vi "PID control fhd.vi"() -> ()   [LabVIEW 2017]
uses:
  <vilib>/Simulation/Scripting/Companion Diagram/SimConfigNode/SimParams.ctl
  <vilib>/Simulation/Scripting/Companion Diagram/SimConfigNode/_simSolvers.ctl
  <vilib>/Simulation/Implementation/Shared/SIMSCR Execution Mode.ctl
  <vilib>/Simulation/Param Hierarchy/Typedefs/SIMPH Param Control Actions.ctl
  <vilib>/Simulation/Implementation/Shared/NILVSim_ParamChanged.vi
  <vilib>/Simulation/Implementation/Shared/NILVSIM_BeginStep.vi
  <vilib>/Simulation/Implementation/Shared/NILVSim_Manager.vi
  <vilib>/Utility/error.llb/Clear Errors.vi
  <vilib>/Simulation/Implementation/Shared/NILVSim_FinalizeModel.vi
  <vilib>/DAQmx/read.llb/DAQmx Read (Counter DBL 1Chan 1Samp).vi
  <vilib>/DAQmx/read.llb/DAQmx Read (Digital Bool 1Line 1Point).vi
  917b7e52-755f-4d44-bea8-9e7c9beac24e.vi
  a58f9967-76f1-4ebc-ad3d-26e75a3ca160.vi
  <vilib>/DAQmx/write.llb/DAQmx Write (Analog DBL 1Chan 1Samp).vi
  <vilib>/DAQmx/create/channels.llb/DAQmx Create Channel (AO-Voltage-Basic).vi
  <vilib>/DAQmx/create/channels.llb/DAQmx Create Channel (DI-Digital Input).vi
  <vilib>/DAQmx/create/channels.llb/DAQmx Create Channel (CI-Count Edges).vi
  <vilib>/Simulation/Implementation/Shared/SIM Unbundle Sim Info.vi
  <vilib>/Simulation/Implementation/Shared/NILVSim_Initialize.vi
  <vilib>/Simulation/Utility/Implementation/NILVSim Get Time and IsAcceptedStep.vi
  <vilib>/Simulation/Implementation/Shared/SIMSH Read Queue.vi
  <vilib>/Simulation/Implementation/Shared/NILVSim_GetModelError.vi
  <vilib>/Simulation/Implementation/Shared/SIM Bundle Sim Info.vi
  <vilib>/DAQmx/miscellaneous.llb/DAQmx Fill In Error Info.vi
  <vilib>/Simulation/Implementation/XNodeFramework/SimXNode/SimX.xnode
  <vilib>/Simulation/Model Libraries/PID/SIM PID (Parallel).vi
  <vilib>/Simulation/Model Libraries/PID/SIM PID.vi
  <vilib>/Simulation/Scripting/Companion Diagram/SimConfigNode/SimDog.xnode
  <vilib>/Simulation/Model Libraries/PID/SIM PID (Academic).vi
  <vilib>/Simulation/Implementation/Shared/NI_SIM_Implementation.lvlib
panel:
  out "Error in x direction":dbl
  out "Error in y direction":dbl
  out "Yerror":dbl
  out "Xerror":dbl
  out "Boolean":bool
  out "Numeric 3":dbl
  out "variable to stop":dbl
  out "index":dbl
  out "x check":dbl
  out "stop":bool
  out "y final check":dbl
  out "y check":dbl
  out "array x Length":dbl
  out "X array":dbl[](array[numeric])
  out "array Y length":dbl
  out "Y array":dbl[](array[numeric])
  out "Numeric y":dbl
  out "Numeric x":dbl
  out "Numeric 2":dbl
  in  "Radius":dbl
  out "led check":bool
  in  "check instruc":bool
  out "down 2":bool
  out "down":bool
  out "right":bool
  out "x entered":dbl
  out "y enetred":dbl
  out "greater -1 x":bool
  out "less 1 x":bool
  out "direction selected":dbl
  out "circle reset":bool
  in  "part circle":T1(ring)=enum."a"
  out "at 2f":bool
  out "Step 2J":bool
  out "Step 2H":bool
  out "Shape drawing steps":enum16{"corner", "1st switch", "reverse"}(ring)
  out "Step 2D":bool
  out "Step 2C":bool
  out "c":bool
  in  "height":dbl
  in  "length":dbl
  in  "part":T2(ring)=enum."a"
  out "Step 2A":bool
  out "Step 2B":bool
  in  "Has encoders been reset?":enum16{"don't reset", "reset"}(ring)
  out "x distance currently being travelled":dbl
  out "y distance currently being travelled":dbl
  out "error calced":dbl
  out "p1 dis 2":dbl
  out "p1 dis":dbl
  out "error y":dbl
  out "calc distance y":dbl
  out "calc distanc x":dbl
  out "error x":dbl
  out "reached y":bool
  out "reached x":bool
  out "Numeric":dbl
  in  "Draw rectangle":bool
  in  "Draw circle":bool
  out "In drawing mode":bool
  in  "Right-Down":bool
  in  "Left-Up":bool
  in  "Left-Down":bool
  in  "Right-Up":bool
  in  "right":bool
  in  "left":bool
  in  "motor 2":dbl(slide)=1.5 scale=-10.0..10.0
  in  "down":bool
  in  "up":bool
  in  "Y Length":dbl=30.0
  in  "X Length":dbl=30.0
  in  "Motor 2 encoder":tag="Dev1/ctr1"
  out "Pulses M2":dbl format="%.2f"
  in  "Motor 1 encoder":tag="Dev1/ctr0"
  out "Pulses M1":dbl format="%.2f"
  out "Right":bool
  out "Bottom":bool
  out "Left":bool
  out "Top":bool
  in  "Switch 4/Line 3":tag="Dev1/port0/line3"
  in  "Switch 3/Line 2":tag="Dev1/port0/line2"
  in  "Switch 2/Line 1":tag="Dev1/port0/line1"
  in  "Switch 1/Line 0":tag="Dev1/port0/line0"
  in  "Motor stop":bool
  in  "Motor 1":tag="Dev1/ao0"
  in  "max Voltage":dbl=10.0
  in  "Min Voltage":dbl=-10.0
  in  "Motor 2":tag="Dev1/ao1"
  in  "motor 1":dbl(slide)=1.5 scale=-10.0..10.0
  in  "stop":bool
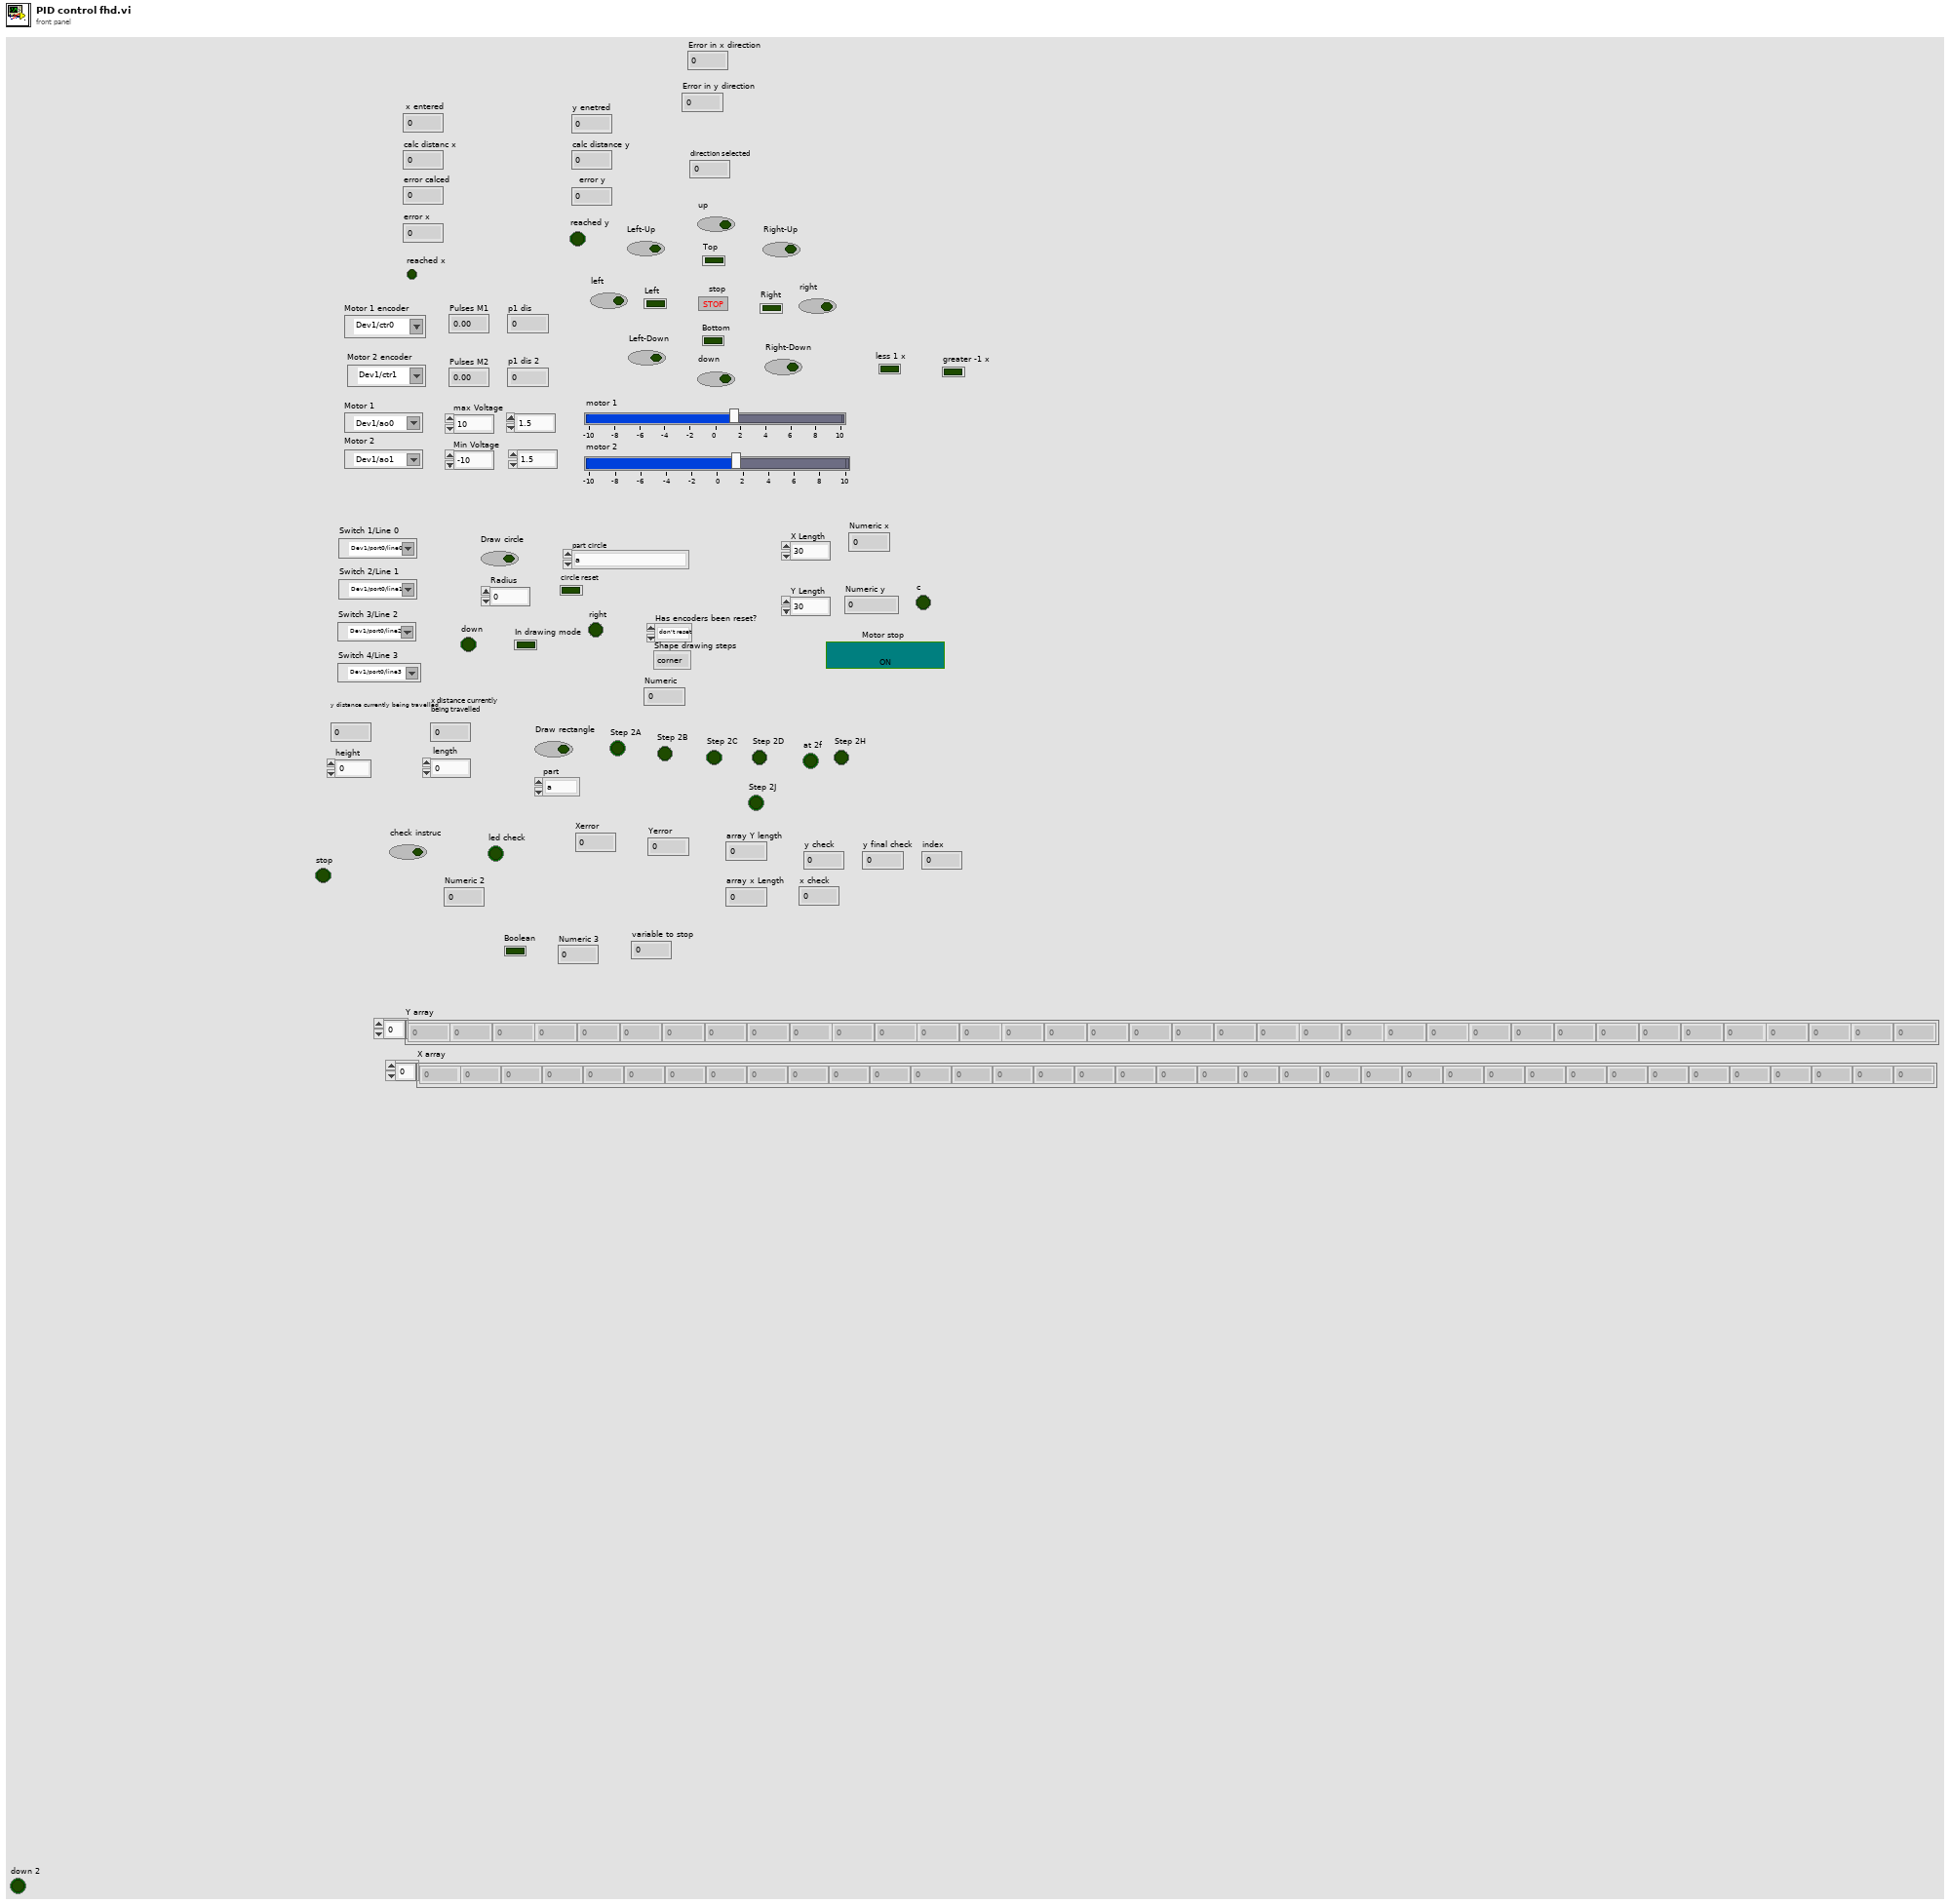
[diagram p1: front panel]
types:
  T1 = enum16{"nothing", "circle", "reset_before_circle", "radius_travel", "going right", "going down", "a"}
  T2 = enum16{"nothing", "j", "i", "h", "g", "f", "e", "d", "c", "b", "a"}
  T3 = enum16{"Simulate to Completion", "Single Time-Step Simulation (Fixed Step Only)"}
  T4 = typedef "SIMSCR Execution Mode.ctl" = enum16{"Simulate to Completion", "Single Time-Step Simulation (Fixed Step Only)"}
  T5 = typedef "SIMPH Param Control Actions.ctl" = enum16{"get params", "set params"}
  T6 = cluster{"SIMSH Sim Time":dbl, "SIM PID Derivative Gain.vi":cluster{"output":dbl}, "SIM PID Derivative Gain.vi - SIMSH":cluster{"SIMSH Sim Time":dbl, "t 3":dbl, "Select 2":cluster{"s? t:f":dbl}, "Equal?":cluster{"x = y?":bool}, "Or":cluster{"x .or. y?":bool}, "Equal To 0?":cluster{"x = 0?":bool}}, "High Frequency [s] (Tf)":dbl, "Gain":cluster{"output":dbl}, "Summation":cluster{"Result":dbl}, "Integral Gain - series.vi":cluster{"output":dbl}, "Integral Gain - series.vi - SIMSH":cluster{"SIMSH Sim Time":dbl, "Select 2":cluster{"s? t:f":dbl}, "integral in gain?":bool, "Integrator":cluster{"output y(t)":dbl}, "Gain 2":cluster{"output":dbl}, "Select":cluster{"s? t:f":dbl}, "Equal To 0?":cluster{"x = 0?":bool}, "Reciprocal":cluster{"1/x":dbl}}}
  T7 = typedef "SimParams.ctl" = cluster{"Initial Time (s)":dbl, "Final Time (s)":dbl, "Step Size (s)":dbl, "ODE Solver":T8, "Minimum Step Size (s)":dbl, "Maximum Step Size (s)":dbl, "Relative Tolerance":dbl, "Absolute Tolerance":dbl, "Software Timing":bool, "Initial Step Size (s)":dbl, "Automatic Fixed Step Size?":bool, "Automatic Discrete Step Size?":bool, "Discrete Step Size (s)":dbl, "Calculate using Time Step":bool, "Solver Wired?":bool, "Prev.Frm.Expected End":u64, "Prev.Frm.Actual End":u64, "Prev.Frm.Finished Late?":bool, "Prev.Iter.Expected End":u64, "Prev.Iter.Actual End":u64, "Prev.Iter.Finished Late?":bool, "Expected Iteration Start":u64, "Actual Iteration Start":u64, "Expected Frame Start":u64, "Actual Frame Start":u64, "Source Name":string, "Name":string, "Period":i64, "Deadline":i64, "Offset":i64, "Start":i64, "Priority":i32, "Timeout":i32, "Processor":i32, "Mode":enum32{"No Change", "Process missed periods, maintain original phase", "Discard missed periods, maintain original phase", "Process missed periods, ignore original phase", "Discard missed periods, ignore original phase"}, "Wakeup reason":enum32{"Normal", "Aborted", "Asynchronous wakeup", "Timing source error", "Timed loop error", "Timeout"}, "Error":errorcluster, "Source Type":string, "Secondary Source Type":string, "Global End Time":u64, "Global Start Time":u64, "Full Solver Reset":bool, "Execution Mode":T4, "Nan/Inf Check":bool, "Custom Solver Library":string, "Solver Is Variable":bool, "custom solver name":string, "Signal Collection Decimation":u32}
  T8 = typedef "_simSolvers.ctl" = enum16{"Runge-Kutta 1 (Euler)", "Runge-Kutta 2", "Runge-Kutta 3", "Runge-Kutta 4", "Runge-Kutta 23 (variable)", "Runge-Kutta 45 (variable)", "BDF (variable)", "Adams-Moulton (variable)", "Rosenbrock (variable)", "Discrete States Only", "SDIRK 4 (variable)", "Radau 5 (variable)", "Radau 9 (variable)", "Radau 13 (variable)", "Radau [Variable Order] (variable)", "Gear's Method (variable)", "Linearizer", "State Query", "Trim Eval", "Custom Solver"}
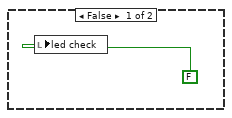
[diagram p2: hidden frame]
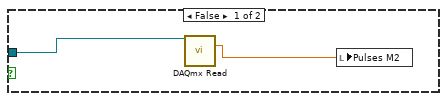
[diagram p3: hidden frame]
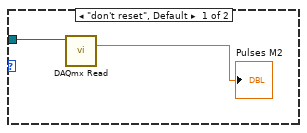
[diagram p4: hidden frame]
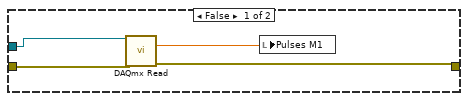
[diagram p5: hidden frame]
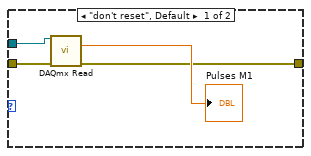
[diagram p6: hidden frame]
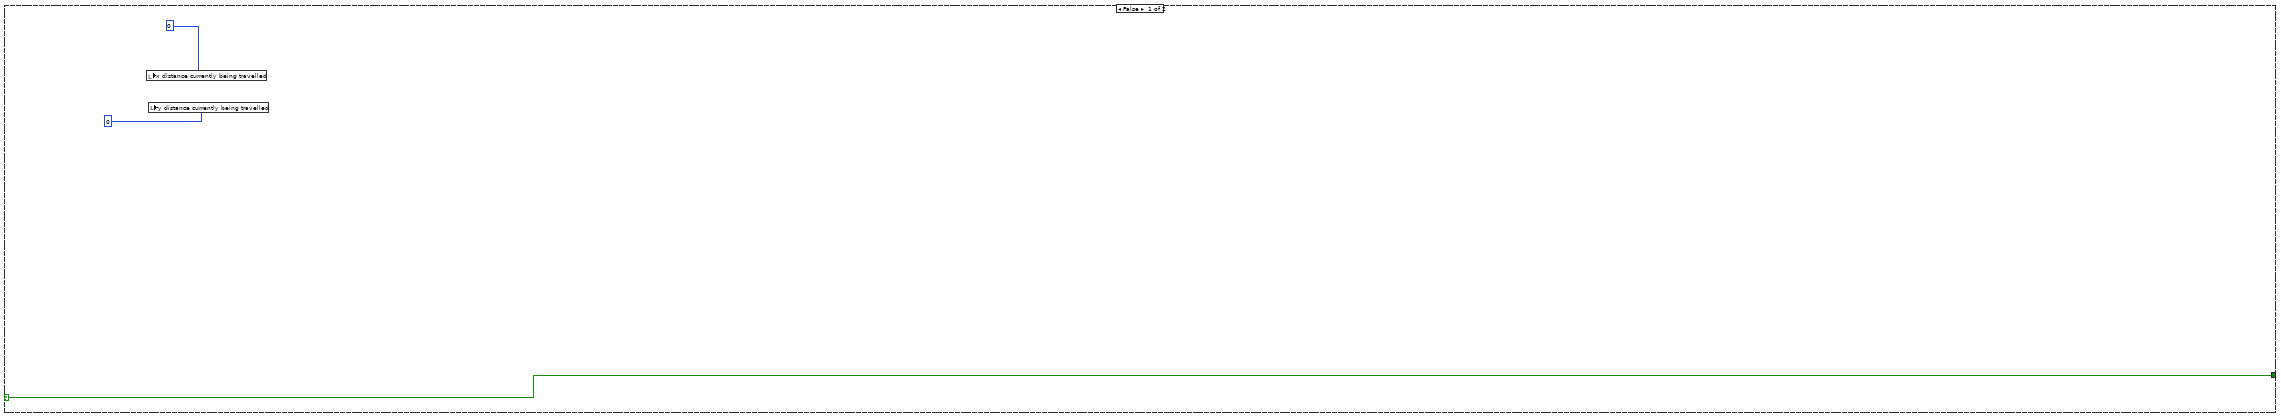
[diagram p7: hidden frame]
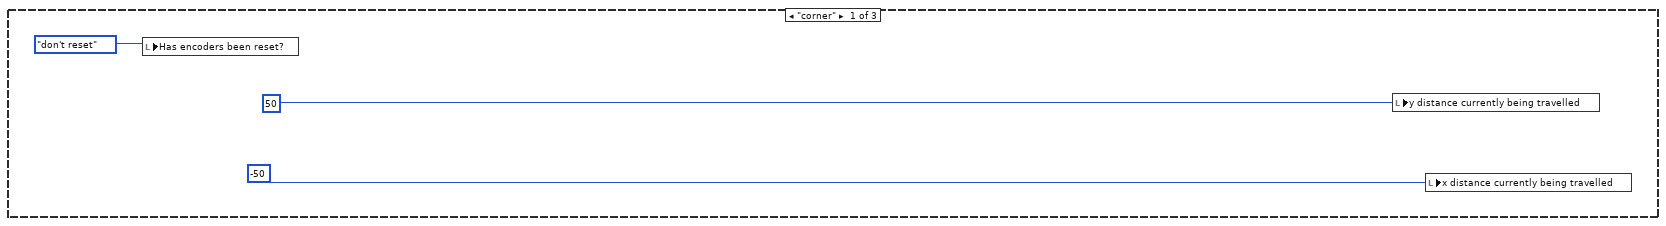
[diagram p8: hidden frame]
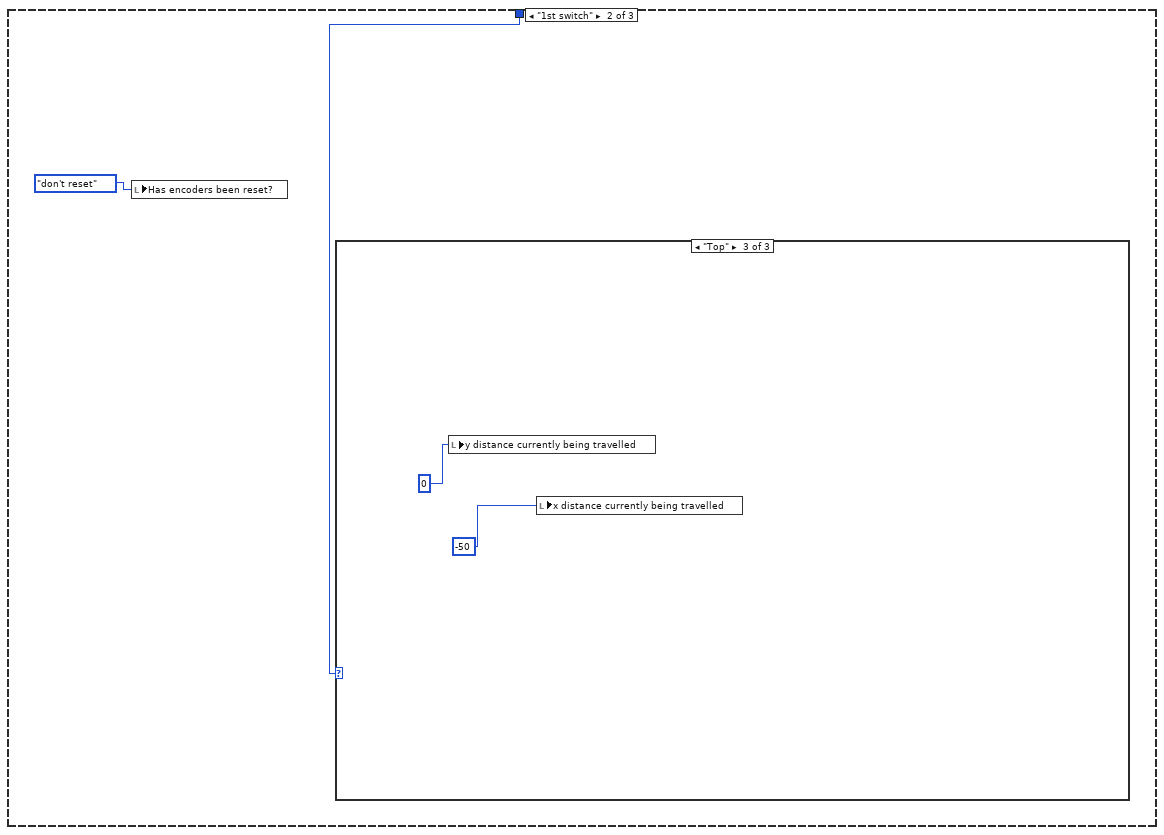
[diagram p9: hidden frame]
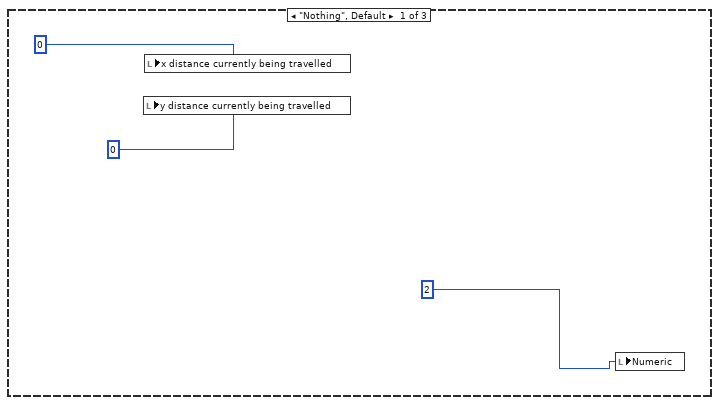
[diagram p10: hidden frame]
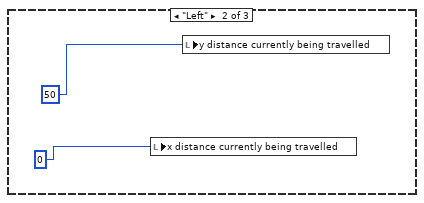
[diagram p11: hidden frame]
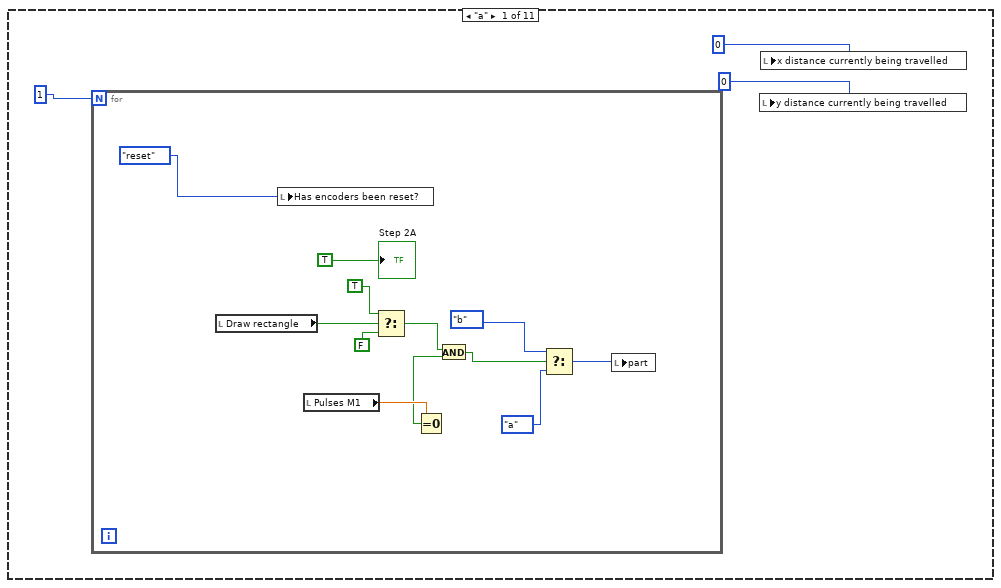
[diagram p12: hidden frame]
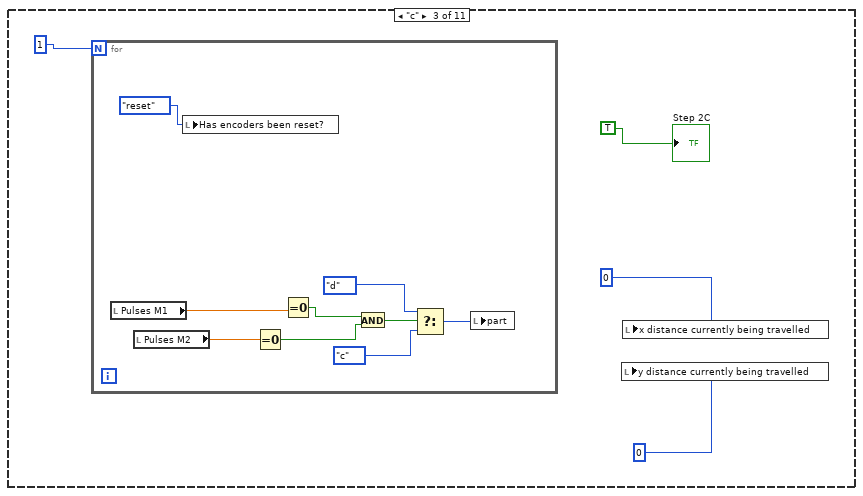
[diagram p13: hidden frame]
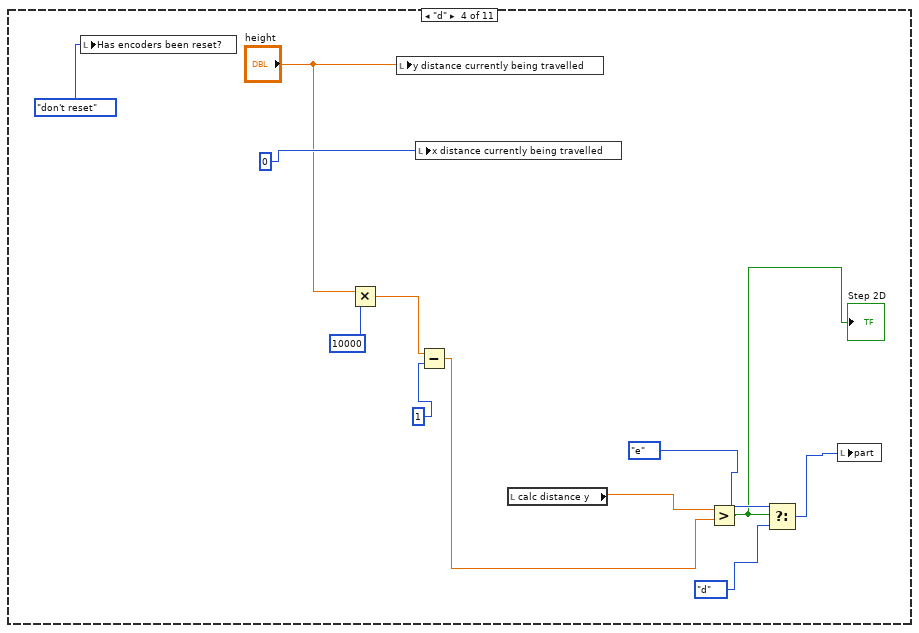
[diagram p14: hidden frame]
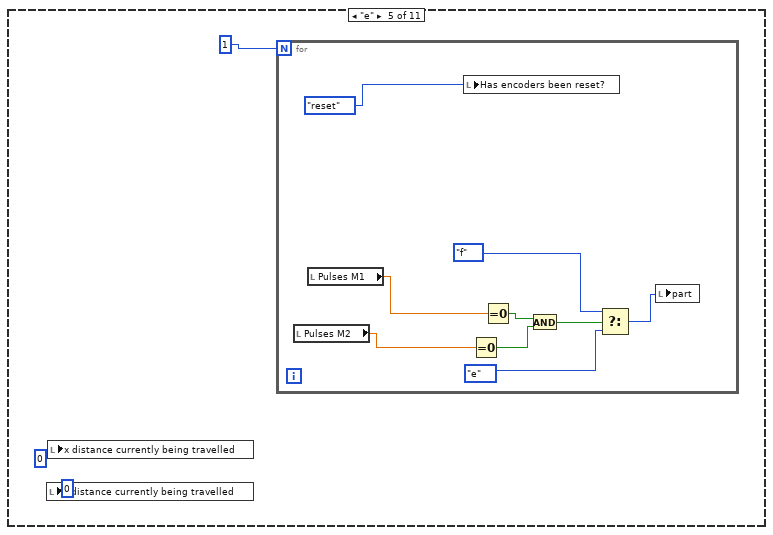
[diagram p15: hidden frame]
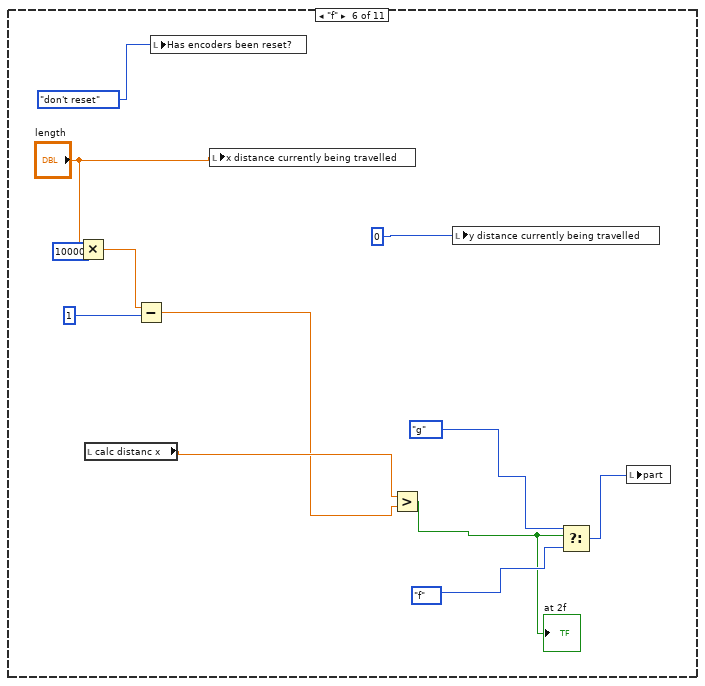
[diagram p16: hidden frame]
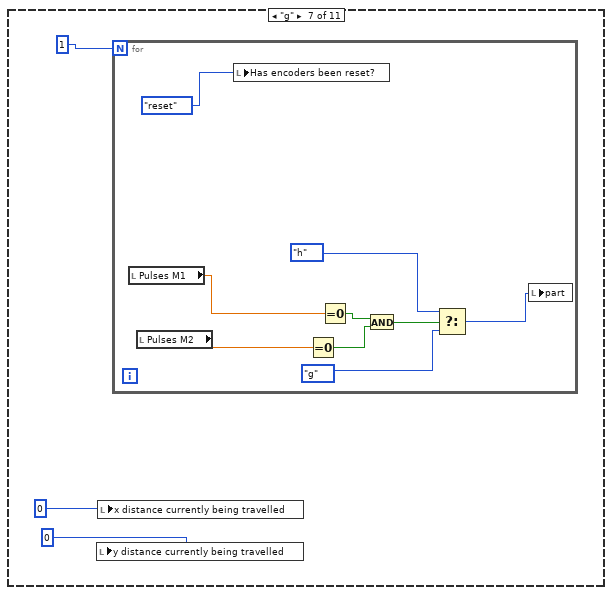
[diagram p17: hidden frame]
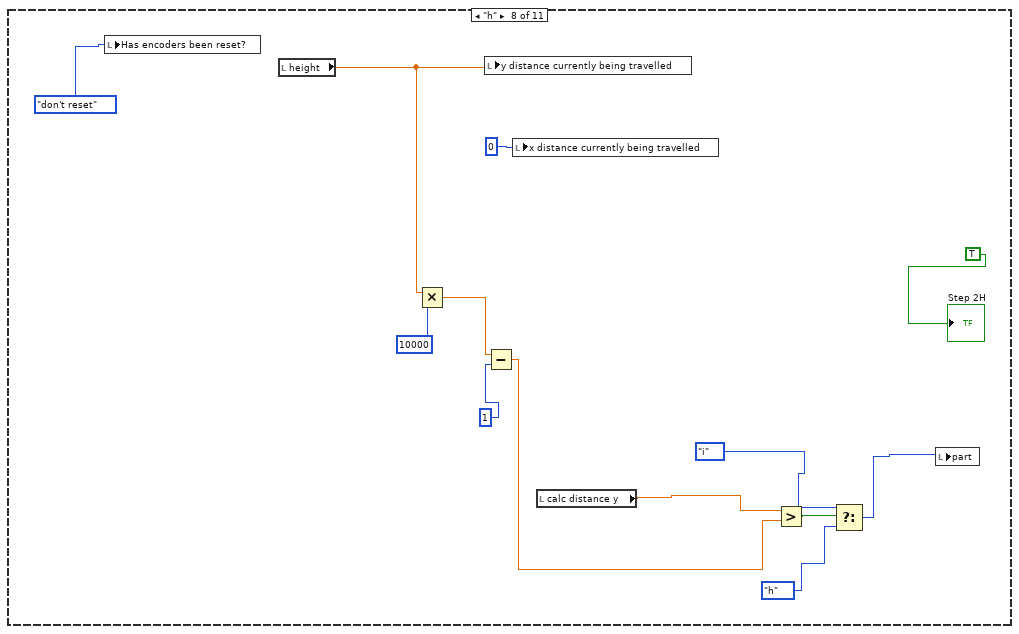
[diagram p18: hidden frame]
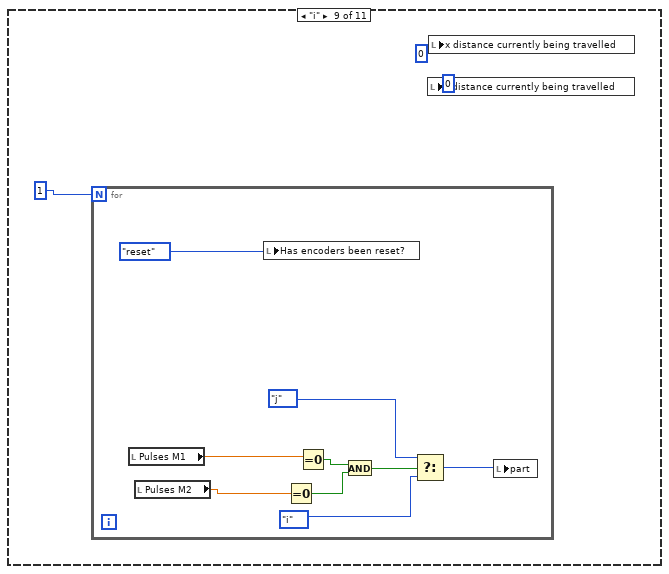
[diagram p19: hidden frame]
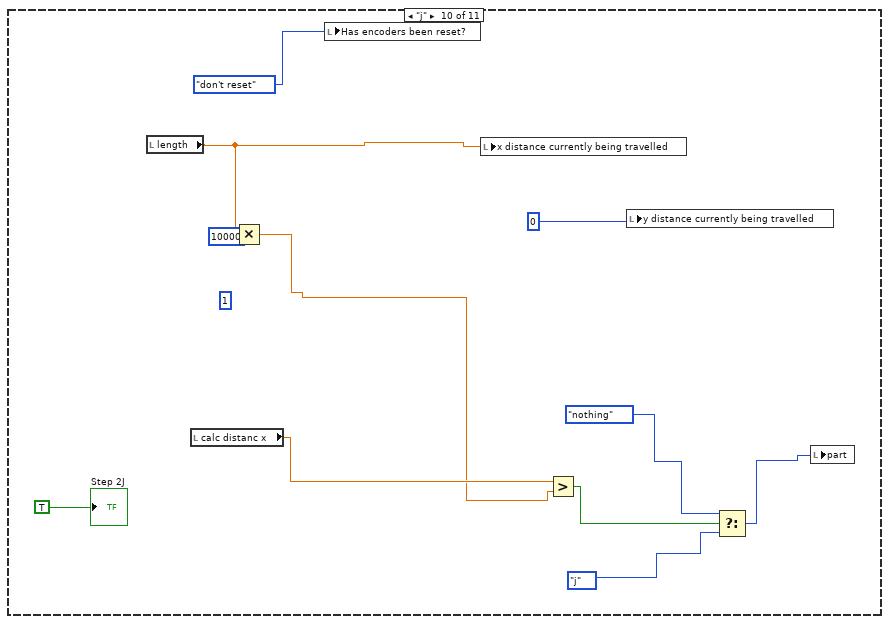
[diagram p20: hidden frame]
diagram:
  n1 = call-poly <vilib>:"DAQmx Create Virtual Channel.vi"("lines"="Switch 1/Line 0") -> ("task out"=w36:refnum<k21>, "error out"=w32:errorcluster)  [unwired: 13 in]
  n2 = call-poly <vilib>:"DAQmx Create Virtual Channel.vi"("lines"="Switch 2/Line 1") -> ("task out"=w35:refnum<k21>, "error out"=w31:errorcluster)  [unwired: 13 in]
  n3 = call-poly <vilib>:"DAQmx Create Virtual Channel.vi"("lines"="Switch 3/Line 2") -> ("task out"=w34:refnum<k21>, "error out"=w30:errorcluster)  [unwired: 13 in]
  n4 = call-poly <vilib>:"DAQmx Create Virtual Channel.vi"("lines"="Switch 4/Line 3") -> ("task out"=w33:refnum<k21>, "error out"=w29:errorcluster)  [unwired: 13 in]
  n5 = call <vilib>:"DAQmx Start Task.vi"("task/channels in"=w36, "error in"=w32) -> ("task out"=w28:refnum<k21>, "error out"=w26:errorcluster)  [unwired: 12 in]
  n6 = call <vilib>:"DAQmx Start Task.vi"("task/channels in"=w35, "error in"=w31) -> ("task out"=w24:refnum<k21>, "error out"=w21:errorcluster)  [unwired: 12 in]
  n7 = call <vilib>:"DAQmx Start Task.vi"("task/channels in"=w34, "error in"=w30) -> ("task out"=w23:refnum<k21>, "error out"=w20:errorcluster)  [unwired: 12 in]
  n8 = call <vilib>:"DAQmx Start Task.vi"("task/channels in"=w33, "error in"=w29) -> ("task out"=w22:refnum<k21>, "error out"=w19:errorcluster)  [unwired: 12 in]
  n9 = call-poly <vilib>:"DAQmx Create Virtual Channel.vi"("maximum value"="max Voltage", "minimum value"="Min Voltage", "physical channels"="Motor 1") -> ("task out"=w46:refnum<k21>, "error out"=w42:errorcluster)  [unwired: 11 in]
  n10 = call-poly <vilib>:"DAQmx Create Virtual Channel.vi"("counter"="Motor 2 encoder") -> ("task out"=w6:refnum<k21>)  [unwired: 13 in, 1 out]
  n11 = call-poly <vilib>:"DAQmx Create Virtual Channel.vi"("maximum value"="max Voltage", "minimum value"="Min Voltage", "physical channels"="Motor 2") -> ("task out"=w49:refnum<k21>, "error out"=w41:errorcluster)  [unwired: 11 in]
  n12 = call-poly <vilib>:"DAQmx Create Virtual Channel.vi"("counter"="Motor 1 encoder") -> ("task out"=w7:refnum<k21>, "error out"=w2:errorcluster)  [unwired: 13 in]
  n13 = call <vilib>:"DAQmx Start Task.vi"("task/channels in"=w6) -> ("task out"=w1:refnum<k21>)  [unwired: 13 in, 1 out]
  n14 = call <vilib>:"DAQmx Start Task.vi"("task/channels in"=w7) -> ("task out"=w3:refnum<k21>)  [unwired: 13 in, 1 out]
  n15 = while {
    tunnel: w49 -> [w228]
    tunnel: [w225] -> w48
    tunnel: w46 -> [w222]
    tunnel: [w221] -> w45
    tunnel: w42 -> [w219]
    tunnel: w41 -> [w218]
    tunnel: w28 -> [w212]
    tunnel: [w211] -> w27
    tunnel: w26 -> [w210]
    tunnel: [w209] -> w25
    tunnel: w24 -> [w208]
    tunnel: w23 -> [w207]
    tunnel: w22 -> [w206]
    tunnel: w21 -> [w205]
    tunnel: w20 -> [w204]
    tunnel: w19 -> [w203]
    tunnel: [w202] -> w18
    tunnel: [w201] -> w17
    tunnel: [w200] -> w16
    tunnel: [w199] -> w15
    tunnel: [w198] -> w14
    tunnel: [w197] -> w13
    tunnel: [w131] -> w10
    tunnel: w3 -> [w133]
    tunnel: w2 -> [w132]
    tunnel: w1 -> [w129]
    stop <- "stop" stop-if-true
    (unwired) TRUE
    n16 = Or(x="Draw circle", y="Draw rectangle") -> (x .or. y?=w141:bool)
    n17 = case shown="True" "check instruc" {
      frame False {
        n18 = local write "led check"(FALSE) -> ()
      }
      frame True {
        n19 = flat-sequence {
          frame #0 {
            n20 = while {
              stop <- w237 stop-if-true
              n21 = for {
                N: 50 -> [_]
                shift-right: [w243] -> w236
                shift-left: _ -> [_]
                tunnel: [w243] -> w231 mode=indexing
                shift-right: [w242] -> w234
                shift-left: _ -> [_]
                tunnel: [w242] -> w232 mode=indexing
                i -> [w245]
                n22 = Multiply(x=2, y=3.141592653589793) -> (x*y=w249:dbl)
                n23 = Increment(x=w245) -> (x+1=w247:i32)
                n24 = Divide(x=w249, y=50) -> (x/y=w251:dbl)
                n25 = Multiply(x=w251, y=w247) -> (x*y=w248:dbl)
                n26 = local write "led check"(TRUE) -> ()
                n27 = local write "Has encoders been reset?"(enum16{"don't reset", "reset"}."don't reset") -> ()
                n28 = Cosine(x=w248) -> (cos(x)=w254:dbl)
                n29 = Sine(x=w248) -> (sin(x)=w255:dbl)
                n30 = Multiply(x=w255, y="Radius") -> (x*y=w243:dbl)
                n31 = Multiply(x=w254, y="Radius") -> (x*y=w242:dbl)
                "Numeric 2" <- w245
              }
              "Numeric y" <- w236
              "Y array" <- w231
              "Numeric x" <- w234
              "X array" <- w232
              n32 = local read "Numeric 2"() -> (w239:dbl)
              n33 = Equal?(x=w239, y=49) -> (x = y?=w237:bool)
              n34 = Array Size(array=w231) -> (size(s)=→"array Y length":i32)
              n35 = Array Size(array=w232) -> (size(s)=→"array x Length":i32)
            }
            n36 = local write "index"(0) -> ()
          }
          frame #1 {
            n37 = flat-sequence {
              tunnel: [w263] -> w259
              tunnel: w257 -> [w263]
              tunnel: w259 -> [w272]
              tunnel: [w284] -> w258
              frame #0 {
                w262 = 1000
                n38 = local read "Y array"() -> (w267:dbl[])
                n39 = local read "X array"() -> (w265:dbl[])
                n40 = local write "variable to stop"(w262) -> ()
                n41 = Index Array(array=w265, index=w263) -> (element=→"x check":dbl)
                n42 = Index Array(array=w267, index=w263) -> (element=→"y check":dbl)
                n43 = local write "Boolean"(FALSE) -> ()
                "Numeric 3" <- w262
                "led check" <- TRUE
              }
              frame #1 {
                n44 = local read "Xerror"() -> (w269:dbl)
                n45 = local read "Yerror"() -> (w271:dbl)
                n46 = Less?(x=w271, y=1) -> (x < y?=w279:bool)
                n47 = Greater?(x=w271, y=-1) -> (0:w278:bool)
                n48 = Less?(x=w269, y=1) -> (x < y?=w275:bool)
                n49 = Greater?(x=w269, y=-1) -> (0:w274:bool)
                n50 = And(x=w279, y=w278) -> (x .and. y?=w277:bool)
                n51 = And(x=w275, y=w274) -> (x .and. y?=w273:bool)
                n52 = And(x=w277, y=w273) -> (x .and. y?=w281:bool)
                "Boolean" <- w281
                n53 = Add(x=1, y=w272) -> (x+y=w282:i32)
                n54 = Select(t=w282, s=w281, f=w272) -> (s? t:f=w284:i32)
                "y final check" <- w284
              }
            }
            n55 = feedback-in #1(w258) -> ()
            n56 = feedback #1() -> (w257:i32)  [unwired: 1 in]
            "index" <- w257
            n57 = local write "Has encoders been reset?"(enum16{"don't reset", "reset"}."don't reset") -> ()
          }
        }
      }
    }
    n58 = local read "calc distance y"() -> (w60:dbl)
    n59 = local read "calc distanc x"() -> (w57:dbl)
    n60 = local read "x entered"() -> (w58:dbl)
    n61 = formula code="if(actual_xLength<0)\nXerror=actual_xLength- desired_xlength;\nelse if (actual_xLength>0)\nXerror=actual_xLength+desired_xlength;"("actual_xLength"=w58, "desired_xlength"=w57) -> ("Xerror"=→"error x":dbl)
    n62 = local read "error y"() -> (w102:dbl)
    n63 = local read "error y"() -> (w101:dbl)
    n64 = local read "error x"() -> (w103:dbl)
    n65 = local read "error y"() -> (w117:dbl)
    n66 = local read "error y"() -> (w114:dbl)
    n67 = local read "error x"() -> (w110:dbl)
    n68 = local read "error x"() -> (w109:dbl)
    n69 = local read "error y"() -> (w118:dbl)
    n70 = local read "error x"() -> (w119:dbl)
    n71 = Less Than 0?(x=w102) -> (x < 0?=w100:bool)
    n72 = Less Than 0?(x=w103) -> (x < 0?=w99:bool)
    n73 = Greater Than 0?(x=w101) -> (x > 0?=w98:bool)
    n74 = Less Than 0?(x=w114) -> (x < 0?=w112:bool)
    n75 = Equal To 0?(x=w119) -> (x = 0?=w113:bool)
    n76 = Greater Than 0?(x=w117) -> (x > 0?=w116:bool)
    n77 = local read "error y"() -> (w95:dbl)
    n78 = local read "error x"() -> (w94:dbl)
    n79 = Greater Than 0?(x=w110) -> (x > 0?=w108:bool)
    n80 = Equal To 0?(x=w118) -> (x = 0?=w107:bool)
    n81 = Less Than 0?(x=w109) -> (x < 0?=w106:bool)
    n82 = And(x=w100, y=w99) -> (x .and. y?=w96:bool)
    n83 = And(x=w99, y=w98) -> (x .and. y?=w97:bool)
    n84 = And(x=w116, y=w113) -> (x .and. y?=w115:bool)
    n85 = And(x=w113, y=w112) -> (x .and. y?=w111:bool)
    n86 = local read "error y"() -> (w90:dbl)
    n87 = And(x=w108, y=w107) -> (x .and. y?=w105:bool)
    n88 = And(x=w107, y=w106) -> (x .and. y?=w104:bool)
    n89 = Greater Than 0?(x=w95) -> (x > 0?=w93:bool)
    n90 = Greater Than 0?(x=w94) -> (x > 0?=w91:bool)
    n91 = Less Than 0?(x=w90) -> (x < 0?=w89:bool)
    n92 = And(x=w93, y=w91) -> (x .and. y?=w92:bool)
    n93 = And(x=w91, y=w89) -> (x .and. y?=w88:bool)
    n94 = Select(t=1, s=w115, f=0) -> (s? t:f=w181:i32)
    n95 = Select(t=10, s=w104, f=0) -> (s? t:f=w179:i32)
    n96 = Select(t=2, s=w111, f=0) -> (s? t:f=w180:i32)
    n97 = Select(t=100, s=w92, f=0) -> (s? t:f=w177:i32)
    n98 = Select(t=200, s=w96, f=0) -> (s? t:f=w176:i32)
    n99 = Select(t=20, s=w105, f=0) -> (s? t:f=w178:i32)
    n100 = Select(t=1000, s=w97, f=0) -> (s? t:f=w175:i32)
    n101 = Select(t=2000, s=w88, f=0) -> (s? t:f=w161:i32)
    n102 = Add(x=w181, y=w180) -> (x+y=w174:i32)
    n103 = Add(x=w179, y=w178) -> (x+y=w173:i32)
    n104 = Add(x=w177, y=w176) -> (x+y=w172:i32)
    n105 = Add(x=w175, y=w161) -> (x+y=w160:i32)
    n106 = local read "y check"() -> (w65:dbl)
    n107 = Add(x=w174, y=w173) -> (x+y=w171:i32)
    n108 = Add(x=w172, y=w160) -> (x+y=w159:i32)
    n109 = call-poly <vilib>:"DAQmx Read.vi"("task/channels in"=w212, "error in"=w210) -> ("task out"=w211:refnum<k21>, "data"=w143:bool, "error out"=w209:errorcluster)  [unwired: 11 in]
    "Top" <- w143
    n110 = call-poly <vilib>:"DAQmx Read.vi"("task/channels in"=w208, "error in"=w205) -> ("task out"=w202:refnum<k21>, "data"=w152:bool, "error out"=w199:errorcluster)  [unwired: 11 in]
    "Bottom" <- w152
    n111 = call-poly <vilib>:"DAQmx Read.vi"("task/channels in"=w207, "error in"=w204) -> ("task out"=w201:refnum<k21>, "data"=w151:bool, "error out"=w198:errorcluster)  [unwired: 11 in]
    "Right" <- w151
    n112 = call-poly <vilib>:"DAQmx Read.vi"("task/channels in"=w206, "error in"=w203) -> ("task out"=w200:refnum<k21>, "data"=w150:bool, "error out"=w197:errorcluster)  [unwired: 11 in]
    "Left" <- w150
    n113 = Add(x=w171, y=w159) -> (x+y=w87:i32)
    "direction selected" <- w87
    n114 = local read "check instruc"() -> (w66:bool)
    n115 = Select(t=w65, s=w66, f="Y Length") -> (s? t:f=w67:dbl)
    n116 = Multiply(x=w67, y=10) -> (x*y=w59:dbl)
    "y enetred" <- w59
    n117 = formula code="if(Ylength<0)\nYerror= Ylength+calculating_y_dis;\nelse if (Ylength>0)\nYerror= Ylength-calculating_y_dis;"("Ylength"=w59, "calculating_y_dis"=w60) -> ("Yerror"=→"error y":dbl)
    n118 = local read "Pulses M1"() -> (w130:dbl)
    n119 = local read "Pulses M2"() -> (w134:dbl)
    n120 = Divide(x=w130, y=52.56) -> (x/y=→"p1 dis":dbl)
    n121 = feedback #2() -> (w79:dbl)  [unwired: 1 in]
    "calc distance y" <- w79
    n122 = formula code="Yerror=( abs(Ylength)-abs(calculating_y_dis));\nif (Yerror<0)\nYerror=0;"("Ylength"=w59, "calculating_y_dis"=w79, "stay"=1) -> ("Yerror"=w64:dbl)
    "Yerror" <- w64
    n123 = Divide(x=w134, y=52.56) -> (x/y=→"p1 dis 2":dbl)
    n124 = formula code="X=((PulseM1/52.56)+(PulseM2/52.56))/2.0;\nY=((PulseM1/52.56)+(PulseM2/52.56))/2.0;"("PulseM1"=w130, "PulseM2"=w134) -> ("X"=w54:dbl, "Y"=w56:dbl)
    "calc distanc x" <- w54
    n125 = feedback-in #2(w56) -> ()
    n126 = local read "check instruc"() -> (w71:bool)
    n127 = local read "x check"() -> (w72:dbl)
    n128 = xnode "PID"("Error"=w64) -> ("Output"=w55:dbl)  [unwired: 2 in, 11 out]
    "Error in y direction" <- w55
    n129 = Select(t=w72, s=w71, f="X Length") -> (s? t:f=w69:dbl)
    n130 = Multiply(x=w69, y=10) -> (x*y=w76:dbl)
    "x entered" <- w76
    n131 = Greater?(x=1, y=w55) -> (0:w85:bool)
    n132 = formula code="Xerror=((abs(desired_xlength))- (abs(actual_xLength)));\nif (Xerror<0)\nXerror=0;"("actual_xLength"=w54, "desired_xlength"=w76, "stay1"=1) -> ("Xerror"=w63:dbl)
    "error calced" <- w63
    "Xerror" <- w63
    n133 = Less?(x=-1, y=w55) -> (x < y?=w83:bool)
    n134 = case shown="2000" w87 {
      tunnel: "motor 1" -> [w1019 w1022 w1025 w1032 w1036 w1040 w1046 w1052 w1058 w1063 w1070]
      tunnel: "motor 2" -> [w1016 w1024 w1027 w1030 w1035 w1038 w1044 w1050 w1056 w1064 w1069]
      tunnel: [w1015 w1024 w1026 w1029 w1035 w1037 w1043 w1049 w1055 w1061 w1068] -> w74
      tunnel: [w1018 w1021 w1025 w1031 w1036 w1039 w1045 w1051 w1057 w1062 w1067] -> w75
      frame 0, Default {
        n135 = Multiply(x=0, y=w1019) -> (x*y=w1018:dbl)
        n136 = Multiply(x=0, y=w1016) -> (x*y=w1015:dbl)
      }
      frame 1 {
        n137 = Multiply(x=-1, y=w1022) -> (x*y=w1021:dbl)
      }
      frame 2 {
        n138 = Multiply(x=-1.003, y=w1027) -> (x*y=w1026:dbl)
      }
      frame 10 {
        n139 = Multiply(x=-1, y=w1032) -> (x*y=w1031:dbl)
        n140 = Multiply(x=-1.1, y=w1030) -> (x*y=w1029:dbl)
      }
      frame 20 {
      }
      frame 100 {
        n141 = Multiply(x=0, y=w1040) -> (x*y=w1039:dbl)
        n142 = Multiply(x=1, y=w1038) -> (x*y=w1037:dbl)
      }
      frame 200 {
        n143 = Multiply(x=0, y=w1046) -> (x*y=w1045:dbl)
        n144 = Multiply(x=-1, y=w1044) -> (x*y=w1043:dbl)
      }
      frame 1000 {
        n145 = Multiply(x=-1, y=w1052) -> (x*y=w1051:dbl)
        n146 = Multiply(x=0, y=w1050) -> (x*y=w1049:dbl)
      }
      frame 2000 {
        n147 = Multiply(x=1, y=w1058) -> (x*y=w1057:dbl)
        n148 = Multiply(x=0, y=w1056) -> (x*y=w1055:dbl)
      }
      frame 4000 {
        n149 = Multiply(x=-1, y=w1063) -> (x*y=w1062:dbl)
        n150 = Multiply(x=0, y=w1064) -> (x*y=w1061:dbl)
      }
      frame 8000 {
        n151 = Multiply(x=-1, y=w1070) -> (x*y=w1067:dbl)
        n152 = Multiply(x=0, y=w1069) -> (x*y=w1068:dbl)
      }
    }
    n153 = And(x=w85, y=w83) -> (x .and. y?=w62:bool)
    "reached y" <- w62
    n154 = xnode "PID 2"("Error"=w63) -> ("Output"=w52:dbl)  [unwired: 2 in, 11 out]
    "Error in x direction" <- w52
    n155 = local read "Numeric"() -> (w123:dbl)
    n156 = Or(x=w152, y=w151) -> (x .or. y?=w195:bool)
    n157 = local read "Draw circle"() -> (w127:bool)
    n158 = local read "Draw rectangle"() -> (w126:bool)
    n159 = And(x=w150, y=w143) -> (x .and. y?=w124:bool)
    n160 = Exclusive Or(1:w143, 2:w150) -> (0:w157:bool)
    n161 = Greater?(x=1, y=w52) -> (0:w80:bool)
    "greater -1 x" <- w80
    n162 = Select(t=1, s=w150, f=0) -> (s? t:f=w142:i32)
    n163 = Select(t=2, s=w143, f=w142) -> (s? t:f=w147:i32)
    n164 = Less?(x=-1, y=w52) -> (x < y?=w81:bool)
    "less 1 x" <- w81
    n165 = And(x=w80, y=w81) -> (x .and. y?=w53:bool)
    "reached x" <- w53
    n166 = Select(t=1, s=w157, f=w123) -> (s? t:f=w156:dbl)
    n167 = Select(t=2, s=w124, f=w156) -> (s? t:f=w154:dbl)
    n168 = Or(x=w127, y=w126) -> (x .or. y?=w128:bool)
    n169 = call "Number To Enum.vim"("number"=w147, "enum type"=enum16{"Nothing", "Left", "Top"}."Nothing") -> ("number as enum"=w144:enum16{"Nothing", "Left", "Top"})
    n170 = case shown="True" w141 {
      selector: w141 -> [w811 w819]
      tunnel: [w811 w819] -> w158
      tunnel: w144 -> [_ w812]
      frame False {
        n171 = local write "x distance currently being travelled"(0) -> ()
        n172 = local write "y distance currently being travelled"(0) -> ()
      }
      frame True {
        n173 = local read "Numeric"() -> (w817:dbl)
        n174 = local read "Shape drawing steps"() -> (w814:enum16{"corner", "1st switch", "reverse"})
        n175 = Equal?(x=w817, y=2) -> (x = y?=w816:bool)
        n176 = Select(t=enum16{"corner", "1st switch", "reverse"}."reverse", s=w816, f=w814) -> (s? t:f=w813:enum16{"corner", "1st switch", "reverse"})
        n177 = case shown="\"reverse\"" w813 {
          tunnel: w812 -> [_ w823 _]
          frame "corner" {
            n178 = local write "Has encoders been reset?"(enum16{"don't reset", "reset"}."don't reset") -> ()
            n179 = local write "y distance currently being travelled"(50) -> ()
            n180 = local write "x distance currently being travelled"(-50) -> ()
          }
          frame "1st switch" {
            n181 = local write "Has encoders been reset?"(enum16{"don't reset", "reset"}."don't reset") -> ()
            n182 = case shown="\"Top\"" w823 {
              frame "Nothing", Default {
                n183 = local write "y distance currently being travelled"(0) -> ()
                n184 = local write "x distance currently being travelled"(0) -> ()
                n185 = local write "Numeric"(2) -> ()
              }
              frame "Left" {
                n186 = local write "x distance currently being travelled"(0) -> ()
                n187 = local write "y distance currently being travelled"(50) -> ()
              }
              frame "Top" {
                n188 = local write "y distance currently being travelled"(0) -> ()
                n189 = local write "x distance currently being travelled"(-50) -> ()
              }
            }
          }
          frame "reverse" {
            n190 = local read "Draw circle"() -> (w832:bool)
            n191 = case shown="False" w832 {
              tunnel: "part" -> [w835 _]
              frame False {
                n192 = case shown="\"b\"" w835 {
                  frame "a" {
                    n193 = for {
                      N: 1 -> [_]
                      n194 = local read "Draw rectangle"() -> (w839:bool)
                      n195 = local write "Has encoders been reset?"(enum16{"don't reset", "reset"}."reset") -> ()
                      n196 = local read "Pulses M1"() -> (w848:dbl)
                      n197 = Select(t=TRUE, s=w839, f=FALSE) -> (s? t:f=w842:bool)
                      n198 = Equal To 0?(x=w848) -> (x = 0?=w841:bool)
                      n199 = And(x=w842, y=w841) -> (x .and. y?=w840:bool)
                      n200 = Select(t=T2."b", s=w840, f=T2."a") -> (s? t:f=w847:T2)
                      n201 = local write "part"(w847) -> ()
                      "Step 2A" <- TRUE
                    }
                    n202 = local write "y distance currently being travelled"(0) -> ()
                    n203 = local write "x distance currently being travelled"(0) -> ()
                  }
                  frame "b" {
                    n204 = local read "calc distance y"() -> (w851:dbl)
                    n205 = local read "calc distanc x"() -> (w852:dbl)
                    n206 = local write "Has encoders been reset?"(enum16{"don't reset", "reset"}."don't reset") -> ()
                    n207 = Greater?(x=w851, y=9000) -> (0:w857:bool)
                    n208 = Greater?(x=w852, y=29000) -> (0:w856:bool)
                    n209 = And(x=w856, y=w857) -> (x .and. y?=w855:bool)
                    "c" <- w855
                    n210 = Select(t=T2."c", s=w855, f=T2."b") -> (s? t:f=w860:T2)
                    n211 = local write "part"(w860) -> ()
                    "x distance currently being travelled" <- 3
                    "y distance currently being travelled" <- 1
                    "Step 2B" <- TRUE
                  }
                  frame "c" {
                    n212 = for {
                      N: 1 -> [_]
                      n213 = local read "Pulses M1"() -> (w876:dbl)
                      n214 = local read "Pulses M2"() -> (w872:dbl)
                      n215 = local write "Has encoders been reset?"(enum16{"don't reset", "reset"}."reset") -> ()
                      n216 = Equal To 0?(x=w872) -> (x = 0?=w870:bool)
                      n217 = Equal To 0?(x=w876) -> (x = 0?=w871:bool)
                      n218 = And(x=w871, y=w870) -> (x .and. y?=w869:bool)
                      n219 = Select(t=T2."d", s=w869, f=T2."c") -> (s? t:f=w875:T2)
                      n220 = local write "part"(w875) -> ()
                    }
                    n221 = local write "y distance currently being travelled"(0) -> ()
                    n222 = local write "x distance currently being travelled"(0) -> ()
                    "Step 2C" <- TRUE
                  }
                  frame "d" {
                    n223 = local write "Has encoders been reset?"(enum16{"don't reset", "reset"}."don't reset") -> ()
                    n224 = Multiply(x="height", y=10000) -> (x*y=w885:dbl)
                    n225 = local write "y distance currently being travelled"("height") -> ()
                    n226 = local write "x distance currently being travelled"(0) -> ()
                    n227 = Subtract(x=w885, y=1) -> (x-y=w882:dbl)
                    n228 = local read "calc distance y"() -> (w887:dbl)
                    n229 = Greater?(x=w887, y=w882) -> (0:w878:bool)
                    "Step 2D" <- w878
                    n230 = Select(t=T2."e", s=w878, f=T2."d") -> (s? t:f=w888:T2)
                    n231 = local write "part"(w888) -> ()
                  }
                  frame "e" {
                    n232 = local write "y distance currently being travelled"(0) -> ()
                    n233 = local write "x distance currently being travelled"(0) -> ()
                    n234 = for {
                      N: 1 -> [_]
                      n235 = local read "Pulses M2"() -> (w894:dbl)
                      n236 = local read "Pulses M1"() -> (w895:dbl)
                      n237 = local write "Has encoders been reset?"(enum16{"don't reset", "reset"}."reset") -> ()
                      n238 = Equal To 0?(x=w894) -> (x = 0?=w900:bool)
                      n239 = Equal To 0?(x=w895) -> (x = 0?=w901:bool)
                      n240 = And(x=w901, y=w900) -> (x .and. y?=w899:bool)
                      n241 = Select(t=T2."f", s=w899, f=T2."e") -> (s? t:f=w893:T2)
                      n242 = local write "part"(w893) -> ()
                    }
                  }
                  frame "f" {
                    n243 = Multiply(x="length", y=10000) -> (x*y=w908:dbl)
                    n244 = local read "calc distanc x"() -> (w911:dbl)
                    n245 = Subtract(x=w908, y=1) -> (x-y=w905:dbl)
                    n246 = local write "Has encoders been reset?"(enum16{"don't reset", "reset"}."don't reset") -> ()
                    n247 = local write "x distance currently being travelled"("length") -> ()
                    n248 = Greater?(x=w911, y=w905) -> (0:w902:bool)
                    "at 2f" <- w902
                    n249 = local write "y distance currently being travelled"(0) -> ()
                    n250 = Select(t=T2."g", s=w902, f=T2."f") -> (s? t:f=w910:T2)
                    n251 = local write "part"(w910) -> ()
                  }
                  frame "g" {
                    n252 = local write "y distance currently being travelled"(0) -> ()
                    n253 = local write "x distance currently being travelled"(0) -> ()
                    n254 = for {
                      N: 1 -> [_]
                      n255 = local read "Pulses M1"() -> (w918:dbl)
                      n256 = local read "Pulses M2"() -> (w917:dbl)
                      n257 = local write "Has encoders been reset?"(enum16{"don't reset", "reset"}."reset") -> ()
                      n258 = Equal To 0?(x=w917) -> (x = 0?=w924:bool)
                      n259 = Equal To 0?(x=w918) -> (x = 0?=w925:bool)
                      n260 = And(x=w925, y=w924) -> (x .and. y?=w923:bool)
                      n261 = Select(t=T2."h", s=w923, f=T2."g") -> (s? t:f=w920:T2)
                      n262 = local write "part"(w920) -> ()
                    }
                  }
                  frame "h" {
                    n263 = local write "Has encoders been reset?"(enum16{"don't reset", "reset"}."don't reset") -> ()
                    n264 = local read "height"() -> (w929:dbl)
                    n265 = Multiply(x=w929, y=10000) -> (x*y=w937:dbl)
                    n266 = local write "y distance currently being travelled"(w929) -> ()
                    n267 = Subtract(x=w937, y=1) -> (x-y=w934:dbl)
                    n268 = local write "x distance currently being travelled"(0) -> ()
                    n269 = local read "calc distance y"() -> (w927:dbl)
                    n270 = Greater?(x=w927, y=w934) -> (0:w938:bool)
                    n271 = Select(t=T2."i", s=w938, f=T2."h") -> (s? t:f=w930:T2)
                    n272 = local write "part"(w930) -> ()
                    "Step 2H" <- TRUE
                  }
                  frame "i" {
                    n273 = for {
                      N: 1 -> [_]
                      n274 = local read "Pulses M1"() -> (w944:dbl)
                      n275 = local read "Pulses M2"() -> (w943:dbl)
                      n276 = local write "Has encoders been reset?"(enum16{"don't reset", "reset"}."reset") -> ()
                      n277 = Equal To 0?(x=w943) -> (x = 0?=w949:bool)
                      n278 = Equal To 0?(x=w944) -> (x = 0?=w950:bool)
                      n279 = And(x=w950, y=w949) -> (x .and. y?=w948:bool)
                      n280 = Select(t=T2."j", s=w948, f=T2."i") -> (s? t:f=w942:T2)
                      n281 = local write "part"(w942) -> ()
                    }
                    n282 = local write "y distance currently being travelled"(0) -> ()
                    n283 = local write "x distance currently being travelled"(0) -> ()
                  }
                  frame "j" {
                    (unwired) 1
                    n284 = local read "length"() -> (w954:dbl)
                    n285 = local read "calc distanc x"() -> (w956:dbl)
                    n286 = Multiply(x=w954, y=10000) -> (x*y=w951:dbl)
                    n287 = local write "Has encoders been reset?"(enum16{"don't reset", "reset"}."don't reset") -> ()
                    n288 = local write "x distance currently being travelled"(w954) -> ()
                    n289 = Greater?(x=w956, y=w951) -> (0:w959:bool)
                    n290 = local write "y distance currently being travelled"(0) -> ()
                    n291 = Select(t=T2."nothing", s=w959, f=T2."j") -> (s? t:f=w955:T2)
                    n292 = local write "part"(w955) -> ()
                    "Step 2J" <- TRUE
                  }
                  frame "nothing" {
                    n293 = local write "y distance currently being travelled"(0) -> ()
                    n294 = local write "x distance currently being travelled"(0) -> ()
                  }
                }
              }
              frame True {
                n295 = case shown="\"radius_travel\"" "part circle" {
                  frame "a" {
                    n296 = for {
                      N: 1 -> [_]
                      n297 = local read "Pulses M1"() -> (w973:dbl)
                      n298 = local read "Pulses M2"() -> (w972:dbl)
                      n299 = Equal To 0?(x=w973) -> (x = 0?=w975:bool)
                      n300 = Equal To 0?(x=w972) -> (x = 0?=w976:bool)
                      n301 = And(x=w975, y=w976) -> (x .and. y?=w974:bool)
                      "circle reset" <- w974
                      n302 = Select(t=T1."going right", s=w974, f=T1."a") -> (s? t:f=w970:T1)
                      n303 = local write "Has encoders been reset?"(enum16{"don't reset", "reset"}."reset") -> ()
                      n304 = local write "part circle"(w970) -> ()
                    }
                    n305 = local write "x distance currently being travelled"(0) -> ()
                    n306 = local write "y distance currently being travelled"(0) -> ()
                  }
                  frame "going down" {
                    n307 = local read "calc distance y"() -> (w985:dbl)
                    n308 = Greater?(x=w985, y=19000) -> (0:w983:bool)
                    n309 = local write "Has encoders been reset?"(enum16{"don't reset", "reset"}."don't reset") -> ()
                    n310 = Select(t=T1."going right", s=w983, f=T1."going down") -> (s? t:f=w980:T1)
                    n311 = local write "y distance currently being travelled"(-2) -> ()
                    n312 = local write "x distance currently being travelled"(0) -> ()
                    n313 = local write "part circle"(w980) -> ()
                    "down" <- TRUE
                  }
                  frame "going right" {
                    n314 = for {
                      N: 1 -> [_]
                      n315 = local read "Pulses M1"() -> (w996:dbl)
                      n316 = local read "Pulses M2"() -> (w995:dbl)
                      n317 = Equal To 0?(x=w996) -> (x = 0?=w998:bool)
                      n318 = Equal To 0?(x=w995) -> (x = 0?=w999:bool)
                      n319 = And(x=w998, y=w999) -> (x .and. y?=w997:bool)
                      n320 = Select(t=T1."radius_travel", s=w997, f=T1."going right") -> (s? t:f=w993:T1)
                      n321 = local write "Has encoders been reset?"(enum16{"don't reset", "reset"}."reset") -> ()
                      n322 = local write "part circle"(w993) -> ()
                    }
                    n323 = local write "x distance currently being travelled"(0) -> ()
                    n324 = local write "y distance currently being travelled"(0) -> ()
                    "right" <- TRUE
                  }
                  frame "radius_travel" {
                    n325 = local read "calc distanc x"() -> (w1002:dbl)
                    n326 = local write "x distance currently being travelled"(-4) -> ()
                    n327 = Greater?(x=w1002, y=39000) -> (0:w1006:bool)
                    n328 = local write "Has encoders been reset?"(enum16{"don't reset", "reset"}."don't reset") -> ()
                    n329 = Select(t=T1."going right", s=w1006, f=T1."going down") -> (s? t:f=w1001:T1)
                    n330 = local write "part circle"(w1001) -> ()
                    "down 2" <- TRUE
                  }
                  frame "reset_before_circle" {
                    n331 = local write "x distance currently being travelled"(0) -> ()
                    n332 = local write "y distance currently being travelled"(0) -> ()
                  }
                  frame "circle" {
                    n333 = local write "x distance currently being travelled"(0) -> ()
                    n334 = local write "y distance currently being travelled"(0) -> ()
                  }
                  frame "nothing" {
                    n335 = local write "x distance currently being travelled"(0) -> ()
                    n336 = local write "y distance currently being travelled"(0) -> ()
                  }
                }
              }
            }
            "Numeric" <- 2
          }
        }
      }
    }
    "In drawing mode" <- w158
    n337 = And(x=w62, y=w53) -> (x .and. y?=w140:bool)
    n338 = Or(x=w195, y=w140) -> (x .or. y?=w194:bool)
    n339 = Or(x=w194, y="Motor stop") -> (x .or. y?=w196:bool)
    n340 = Or(x=w196, y="stop") -> (x .or. y?=w216:bool)
    n341 = Select(t=0.0, s=w216, f=w74) -> (s? t:f=w213:dbl)
    n342 = call-poly <vilib>:"DAQmx Write.vi"("task/channels in"=w222, "data"=w213, "error in"=w219) -> ("task out"=w223:refnum<k21>, "error out"=w224:errorcluster)  [unwired: 10 in, 1 out]
    n343 = Select(t=0.0 ("s? t:f"), s=w216, f=w75) -> (s? t:f=w214:dbl)
    n344 = call-poly <vilib>:"DAQmx Write.vi"("task/channels in"=w228, "data"=w214, "error in"=w218) -> ("task out"=w227:refnum<k21>, "error out"=w226:errorcluster)  [unwired: 10 in, 1 out]
    n345 = call <vilib>:"DAQmx Wait Until Done.vi"("task/channels in"=w227, "error in"=w226) -> ("error out"=w225:errorcluster)  [unwired: 12 in, 1 out]
    n346 = call <vilib>:"DAQmx Wait Until Done.vi"("task/channels in"=w223, "error in"=w224) -> ("error out"=w221:errorcluster)  [unwired: 12 in, 1 out]
    n347 = case shown="True" w128 {
      tunnel: w129 -> [w286 w287]
      frame False {
        n348 = call-poly <vilib>:"DAQmx Read.vi"("task/channels in"=w286) -> ("data"=w285:dbl)  [unwired: 12 in, 2 out]
        n349 = local write "Pulses M2"(w285) -> ()
      }
      frame True {
        n350 = local read "Has encoders been reset?"() -> (w288:enum16{"don't reset", "reset"})
        n351 = case shown="\"reset\"" w288 {
          tunnel: w287 -> [w290 w293]
          frame "don't reset", Default {
            n352 = call-poly <vilib>:"DAQmx Read.vi"("task/channels in"=w290) -> ("data"=→"Pulses M2":dbl)  [unwired: 12 in, 2 out]
          }
          frame "reset" {
            n353 = call <vilib>:"DAQmx Stop Task.vi"("task/channels in"=w293) -> ("task out"=w292:refnum<k21>)  [unwired: 13 in, 1 out]
            n354 = call <vilib>:"DAQmx Start Task.vi"("task/channels in"=w292) -> ("task out"=w294:refnum<k21>)  [unwired: 13 in, 1 out]
            n355 = call-poly <vilib>:"DAQmx Read.vi"("task/channels in"=w294) -> ("data"=w291:dbl)  [unwired: 12 in, 2 out]
            n356 = local write "Pulses M2"(w291) -> ()
          }
        }
      }
    }
    n357 = call "Number To Enum.vim"("number"=w154, "enum type"=enum16{"corner", "1st switch", "reverse"}."corner") -> ("number as enum"=→"Shape drawing steps":enum16{"corner", "1st switch", "reverse"})
    n358 = case shown="True" w128 {
      tunnel: w133 -> [w297 w302]
      tunnel: w132 -> [w298 w301]
      tunnel: [w295 w300] -> w131
      frame False {
        n359 = call-poly <vilib>:"DAQmx Read.vi"("task/channels in"=w297, "error in"=w298) -> ("data"=w296:dbl, "error out"=w295:errorcluster)  [unwired: 11 in, 1 out]
        n360 = local write "Pulses M1"(w296) -> ()
      }
      frame True {
        n361 = case shown="\"reset\"" "Has encoders been reset?" {
          tunnel: w302 -> [w306 w313]
          tunnel: w301 -> [w305 w312]
          tunnel: [w303 w314] -> w300
          frame "don't reset", Default {
            n362 = call-poly <vilib>:"DAQmx Read.vi"("task/channels in"=w306, "error in"=w305) -> ("data"=→"Pulses M1":dbl, "error out"=w303:errorcluster)  [unwired: 11 in, 1 out]
          }
          frame "reset" {
            n363 = call <vilib>:"DAQmx Stop Task.vi"("task/channels in"=w313, "error in"=w312) -> ("task out"=w311:refnum<k21>, "error out"=w310:errorcluster)  [unwired: 12 in]
            n364 = call <vilib>:"DAQmx Start Task.vi"("task/channels in"=w311, "error in"=w310) -> ("task out"=w309:refnum<k21>, "error out"=w308:errorcluster)  [unwired: 12 in]
            n365 = call-poly <vilib>:"DAQmx Read.vi"("task/channels in"=w309, "error in"=w308) -> ("data"=w307:dbl, "error out"=w314:errorcluster)  [unwired: 11 in, 1 out]
            n366 = local write "Pulses M1"(w307) -> ()
          }
        }
      }
    }
  }
  n367 = invoke on="motor 1" class="Slide (strict)" method="Reinit To Default"() -> ()  [unwired: 3 in, 3 out]
  n368 = invoke on="Numeric 2" class="DigNum (strict)" method="Reinit To Default"() -> ()  [unwired: 3 in, 3 out]
  n369 = invoke on="index" class="DigNum (strict)" method="Reinit To Default"() -> ()  [unwired: 3 in, 3 out]
  n370 = invoke on="y final check" class="DigNum (strict)" method="Reinit To Default"() -> ()  [unwired: 3 in, 3 out]
  n371 = call <vilib>:"Simple Error Handler.vi"("error source (\" \")"="you messed up" ("error source (\" \")"), "error in (no error)"=w48) -> ()  [unwired: 3 in, 5 out]
  n372 = call <vilib>:"Simple Error Handler.vi"("error source (\" \")"="you messed up" ("error source (\" \")"), "error in (no error)"=w45) -> ()  [unwired: 3 in, 5 out]
  n373 = call <vilib>:"DAQmx Clear Task.vi"("task in"=w27, "error in"=w25) -> ()  [unwired: 13 in, 1 out]
  n374 = call <vilib>:"DAQmx Clear Task.vi"("task in"=w17, "error in"=w14) -> ()  [unwired: 13 in, 1 out]
  n375 = call <vilib>:"DAQmx Clear Task.vi"("task in"=w18, "error in"=w15) -> ("error out"=w12:errorcluster)  [unwired: 13 in]
  n376 = call <vilib>:"DAQmx Clear Task.vi"("task in"=w16, "error in"=w13) -> ()  [unwired: 13 in, 1 out]
  n377 = call <vilib>:"Simple Error Handler.vi"("error in (no error)"=w12) -> ()  [unwired: 4 in, 5 out]
  n378 = call <vilib>:"Simple Error Handler.vi"("error source (\" \")"="you messed up" ("error source (\" \")"), "error in (no error)"=w10) -> ()  [unwired: 3 in, 5 out]
